vi "Manual Mode Dialog.vi"(7 "Console Log in":refnum<class "Console Log.lvclass">, 8 "error in":errorcluster, 11 "Gantry in":refnum<class "Gantry Class.lvclass">) -> (0 "error out":errorcluster, 3 "Gantry out":refnum<class "Gantry Class.lvclass">, 5 "Console Log out":refnum<class "Console Log.lvclass">)   [LabVIEW 2011]
uses:
  Shared Components/Gantry Class/Gantry Class.lvclass
  Console Log/Console Log.lvclass
  <vilib>/Native 3D Graph/xcontrol/3DPC_SurfacePlot.xctl
  Shared Components/Config Manager Class/Type Definitions/Camera Enum.ctl
  Shared Components/Vec3d Class/Vec3d Class.lvclass
panel:
  out "Gantry History":refnum<class "Base Datatype.lvclass">[](xcontrol)
  in  "Vacuum Control":T1
  in  "Dispenser":bool
  in  "MPG":bool
  out "Current Location":cluster{"X":dbl, "Y":dbl, "Z":dbl} {"Z" format="%7_6f"; "Y" format="%7_6f"; "X" format="%7_6f"}
  out "Preview":T2(plugin-control)
  in  "Exit Manual Mode":bool
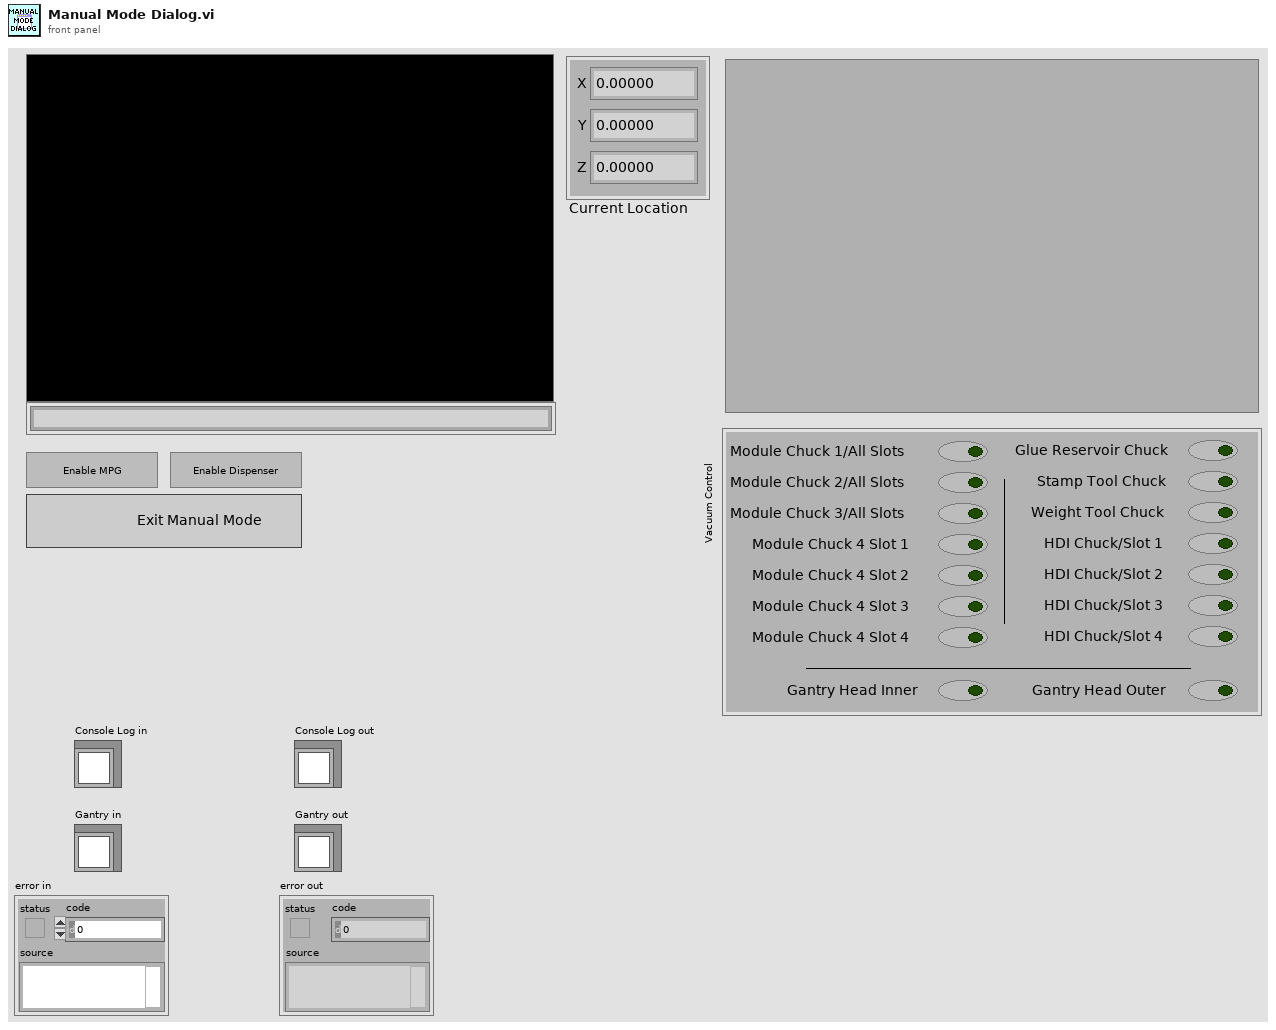
[diagram p1: front panel]
types:
  T1 = cluster{"Module Chuck 1/All Slots":bool, "Module Chuck 2/All Slots":bool, "Module Chuck 3/All Slots":bool, "Module Chuck 4 Slot 1":bool, "Module Chuck 4 Slot 2":bool, "Module Chuck 4 Slot 3":bool, "Module Chuck 4 Slot 4":bool, "Glue Reservoir Chuck":bool, "Stamp Tool Chuck":bool, "Weight Tool Chuck":bool, "HDI Chuck/Slot 1":bool, "HDI Chuck/Slot 2":bool, "HDI Chuck/Slot 3":bool, "HDI Chuck/Slot 4":bool, "Gantry Head Inner":bool, "Gantry Head Outer":bool}
  T2 = typedef "IMAQ Image.ctl" = refnum<image>
  T3 = typedef "Camera Enum.ctl" = enum16{"GANTRY HEAD", "NEEDLE CALIBRATION X", "NEEDLE CALIBRATION Y"}
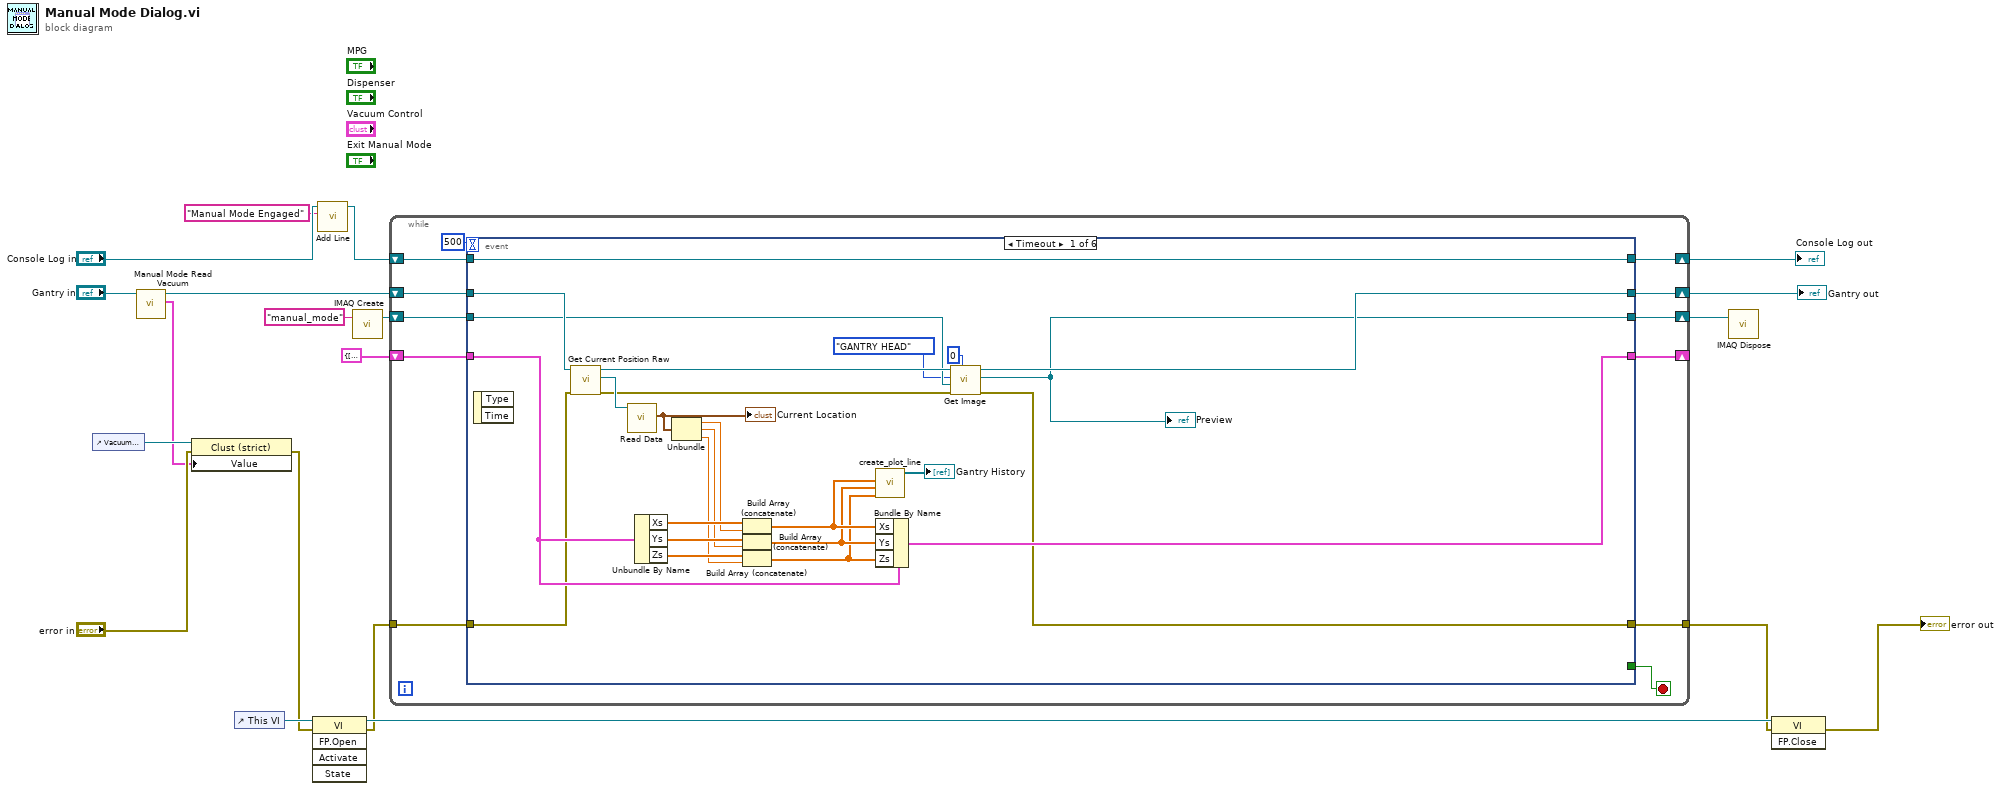
[diagram p0: block diagram]
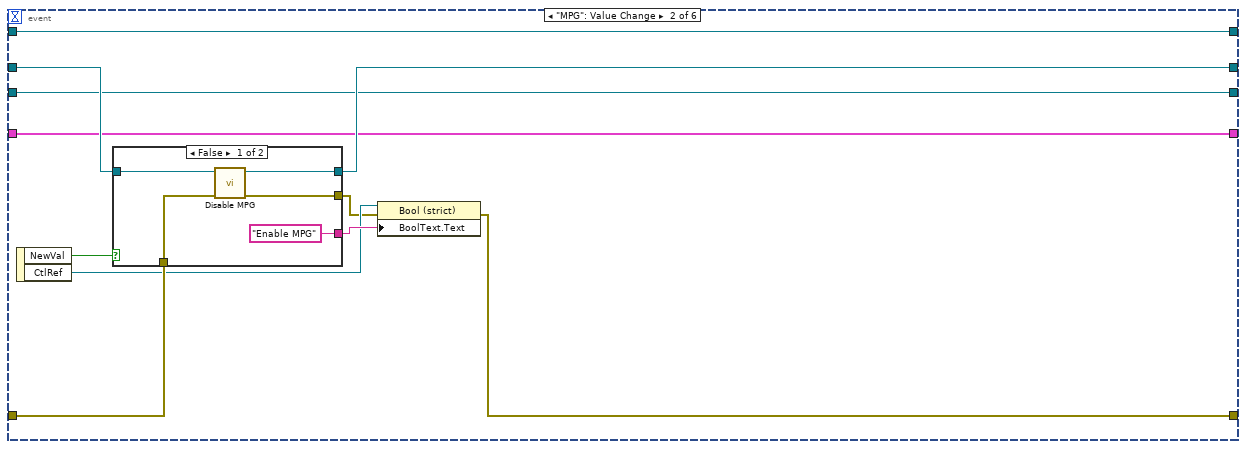
[diagram p2: hidden frame]
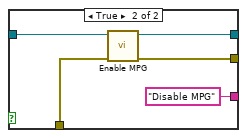
[diagram p3: hidden frame]
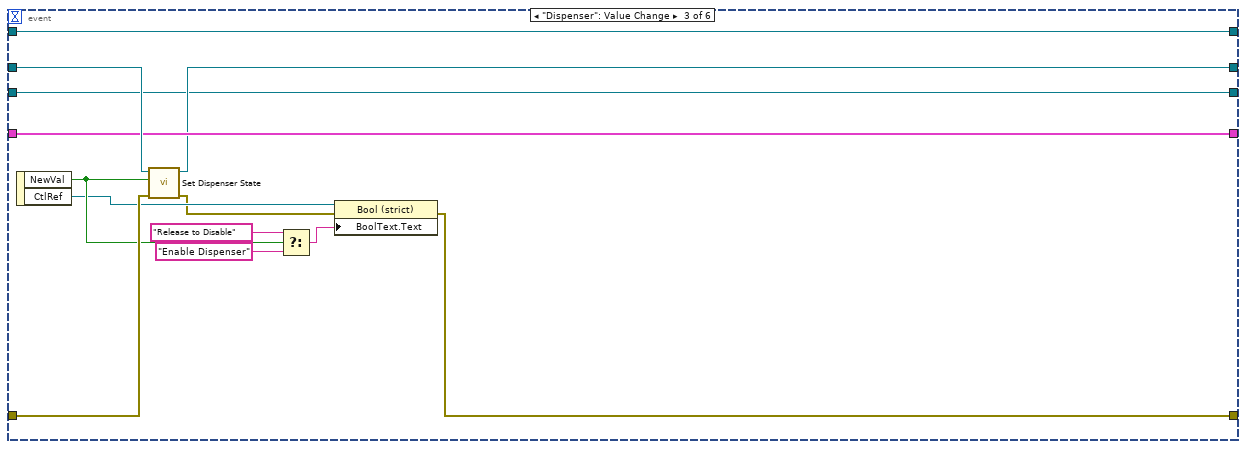
[diagram p4: hidden frame]
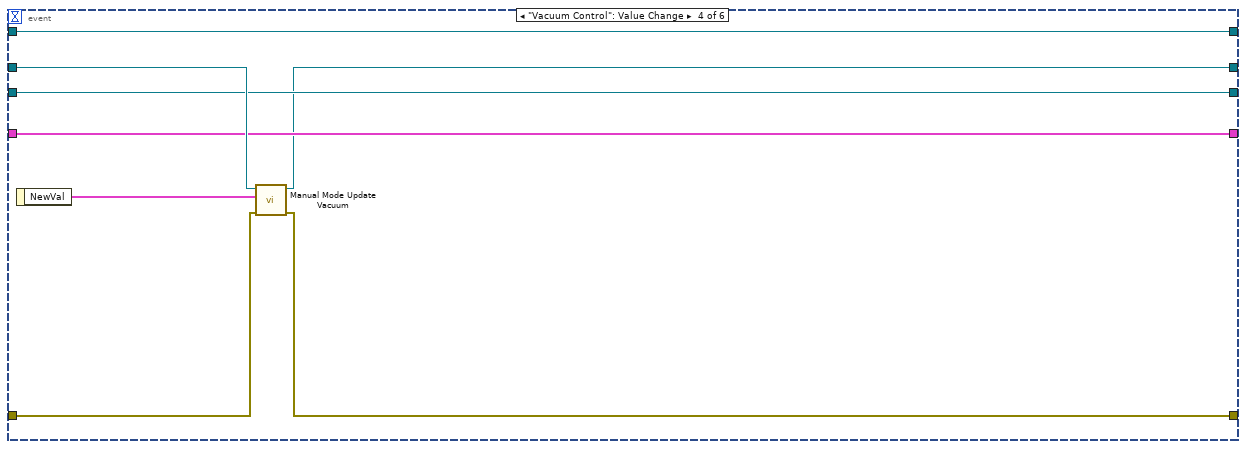
[diagram p5: hidden frame]
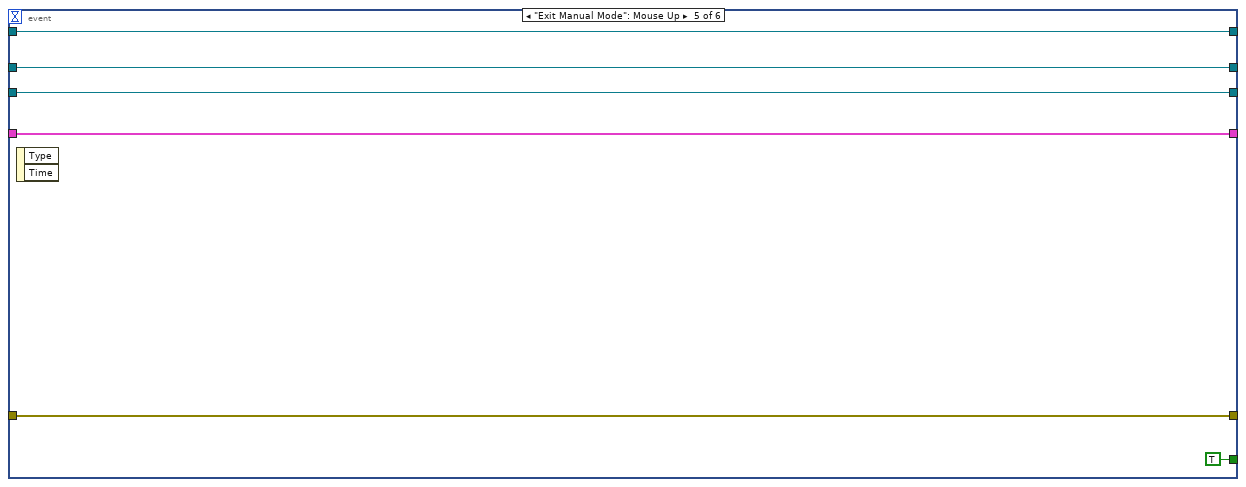
[diagram p6: hidden frame]
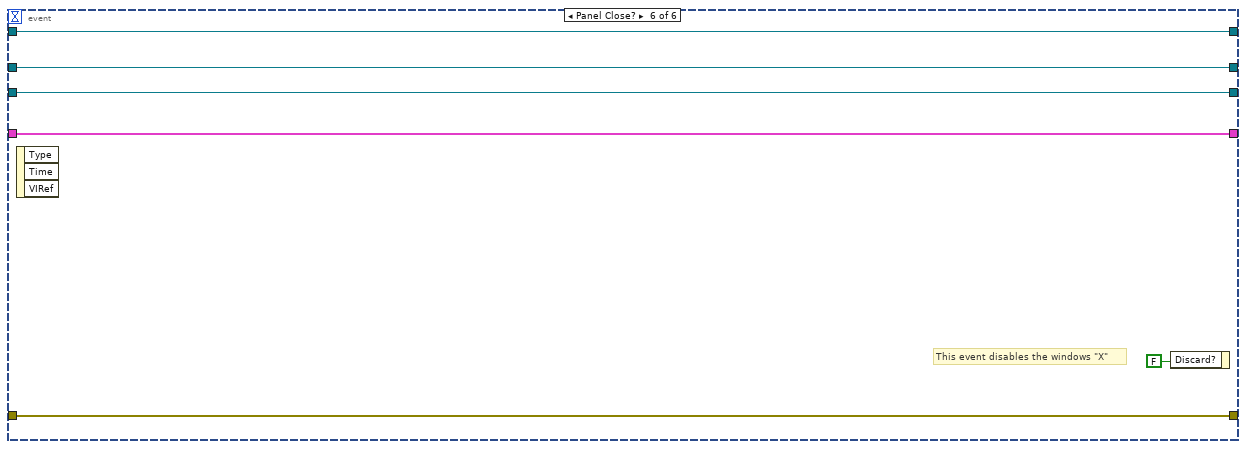
[diagram p7: hidden frame]
diagram:
  n1 = control-ref of="Vacuum Control"() -> (w4:refnum<vi>)
  n2 = call "Manual Mode Read Vacuum.vi"("Gantry in"="Gantry in") -> ("Vacuum Status"=w1:T1, "Gantry out"=w5:refnum<class "Gantry Class.lvclass">)  [unwired: 8 in, 1 out]
  n3 = property class="Clust (strict)"(reference=w4, error in="error in", "Value"=w1) -> (error out=w2:errorcluster)  [unwired: 1 out]
  n4 = control-ref of="This VI"() -> (w20:refnum<vi>)
  n5 = invoke class="VI" method="FP.Open"(reference=w20, error in=w2) -> (reference out=w19:refnum<vi>, error out=w17:errorcluster)  [unwired: 3 in, 3 out]
  n6 = call "Add Line.vi"("String"="Manual Mode Engaged", "Console Log in"="Console Log in") -> ("Console Log out"=w11:refnum<class "Console Log.lvclass">)  [unwired: 8 in, 1 out]
  n7 = call "IMAQ Create"("Image Name"="manual_mode") -> ("New Image"=w8:T2)  [unwired: 4 in, 1 out]
  n8 = while {
    tunnel: w17 -> [w29]
    tunnel: [w30] -> w16
    shift-right: [w25] -> _
    shift-left: cluster{"Xs":dbl[], "Ys":dbl[], "Zs":dbl[]} {"Xs"=[], "Ys"=[], "Zs"=[]} -> [w28]
    shift-right: [w24] -> w14
    shift-left: w11 -> [w27]
    shift-right: [w21] -> w7
    shift-left: w8 -> [w22]
    shift-right: [w23] -> w13
    shift-left: w5 -> [w26]
    stop <- w31 stop-if-true
    n9 = event shown="[0] Timeout" {
      selector: _ -> [_ _ _ _ _ _]
      dyn-events: _ -> [_ _ _ _ _ _]
      timeout: 500 -> [_ _ _ _ _ _]
      tunnel: [_ _ _ _ TRUE _] -> w31
      tunnel: [w36 w60 w79 w92 w105 w110] -> w30
      tunnel: w29 -> [w39 w64 w87 w93 w105 w110]
      tunnel: w28 -> [w49 w59 w90 w97 w101 w106]
      tunnel: w27 -> [w47 w68 w88 w99 w103 w109]
      tunnel: w26 -> [w57 w67 w91 w98 w102 w108]
      tunnel: [w48 w59 w90 w97 w101 w106] -> w25
      tunnel: [w47 w68 w88 w99 w103 w109] -> w24
      tunnel: [w40 w66 w89 w95 w102 w108] -> w23
      tunnel: w22 -> [w37 w58 w86 w96 w100 w107]
      tunnel: [w35 w58 w86 w96 w100 w107] -> w21
      event Timeout {
        n10 = event-data() -> ()  [unwired: 1 in, 2 out]
        n11 = call-dynamic "Get Current Position Raw.vi"("error in"=w39, "Gantry in"=w57) -> ("error out"=w38:errorcluster, "Vec3d Class out"=w56:refnum<class "Vec3d Class.lvclass">, "Gantry out"=w41:refnum<class "Gantry Class.lvclass">)  [unwired: 7 in]
        n12 = call-dynamic "Read Data.vi"("Vec3d Class in"=w56) -> ("Data"=w46:cluster{"X":dbl, "Y":dbl, "Z":dbl})  [unwired: 8 in, 2 out]
        "Current Location" <- w46
        n13 = Unbundle By Name(w49) -> ("Xs"=w55:dbl[], "Ys"=w54:dbl[], "Zs"=w53:dbl[])
        n14 = Unbundle(w46) -> ("X"=w50:dbl, "Y"=w51:dbl, "Z"=w52:dbl)
        n15 = Build Array (concatenate)(w55, w50) -> (w44:dbl[])
        n16 = Build Array (concatenate)(w54, w51) -> (w43:dbl[])
        n17 = Build Array (concatenate)(w53, w52) -> (w42:dbl[])
        n18 = call <vilib>:"create_plot_line.vi"("z vector"=w42, "y vector"=w43, "x vector"=w44) -> ("plots out"=→"Gantry History":refnum<class "Base Datatype.lvclass">[])  [unwired: 2 in, 6 out]
        n19 = Bundle By Name(cluster=w49, "Xs"=w44, "Ys"=w43, "Zs"=w42) -> (w48:cluster{"Xs":dbl[], "Ys":dbl[], "Zs":dbl[]})
        n20 = call-dynamic "Get Image.vi"("Delay(milliseconds)"=0, "error in"=w38, "Image In"=w37, "Camera Name"=Camera_Enum."GANTRY HEAD", "Gantry in"=w41) -> ("error out"=w36:errorcluster, "Image Out"=w35:T2, "Gantry out"=w40:refnum<class "Gantry Class.lvclass">)  [unwired: 3 in, 1 out]
        "Preview" <- w35
      }
      event "MPG": Value Change {
        n21 = event-data() -> ("NewVal"=w65:bool, "CtlRef"=w62:refnum<vi>)  [unwired: 1 in]
        n22 = case shown="False" w65 {
          tunnel: w67 -> [w73 w78]
          tunnel: [w72 w77] -> w66
          tunnel: w64 -> [w71 w76]
          tunnel: [w70 w75] -> w61
          tunnel: ["Enable MPG" ("Boolean Text.Text") "Disable MPG" ("Boolean Text.Text")] -> w63
          frame False {
            n23 = call-dynamic "Disable MPG.vi"("error in"=w71, "Gantry in"=w73) -> ("error out"=w70:errorcluster, "Gantry out"=w72:refnum<class "Gantry Class.lvclass">)  [unwired: 8 in]
          }
          frame True {
            n24 = call-dynamic "Enable MPG.vi"("error in"=w76, "Gantry in"=w78) -> ("error out"=w75:errorcluster, "Gantry out"=w77:refnum<class "Gantry Class.lvclass">)  [unwired: 8 in]
          }
        }
        n25 = property class="Bool (strict)"(reference=w62, error in=w61, "BoolText.Text"=w63) -> (error out=w60:errorcluster)  [unwired: 1 out]
      }
      event "Dispenser": Value Change {
        n26 = event-data() -> ("NewVal"=w85:bool, "CtlRef"=w84:refnum<vi>)  [unwired: 1 in]
        n27 = call-dynamic "Set Dispenser State.vi"("error in"=w87, "On/Off"=w85, "Gantry in"=w91) -> ("error out"=w83:errorcluster, "Gantry out"=w89:refnum<class "Gantry Class.lvclass">)  [unwired: 7 in]
        n28 = Select(t="Release to Disable", s=w85, f="Enable Dispenser") -> (s? t:f=w80:string)
        n29 = property class="Bool (strict)"(reference=w84, error in=w83, "BoolText.Text"=w80) -> (error out=w79:errorcluster)  [unwired: 1 out]
      }
      event "Vacuum Control": Value Change {
        n30 = event-data() -> ("NewVal"=w94:T1)  [unwired: 1 in]
        n31 = call "Manual Mode Update Vacuum.vi"("error in"=w93, "Vacuum Status"=w94, "Gantry in"=w98) -> ("error out"=w92:errorcluster, "Gantry out"=w95:refnum<class "Gantry Class.lvclass">)  [unwired: 7 in]
      }
      event "Exit Manual Mode": Mouse Up {
        n32 = event-data() -> ()  [unwired: 1 in, 2 out]
      }
      event Panel Close? {
        # "This event disables the windows \"X\""
        n33 = event-data() -> ()  [unwired: 1 in, 3 out]
        n34 = event-data("Discard?"=FALSE) -> ()  [unwired: 1 in, 1 out]
      }
    }
  }
  "Gantry out" <- w13
  "Console Log out" <- w14
  n35 = call "IMAQ Dispose"("Image"=w7) -> ()  [unwired: 5 in, 1 out]
  n36 = invoke class="VI" method="FP.Close"(reference=w19, error in=w16) -> (error out=→"error out":errorcluster)  [unwired: 1 in, 2 out]
